vi "equ2hor.vi"(4 "deltat":dbl[unit], 5 "TimeStamp [UT]":timestamp format="%<%H:%M:%S%6u\n%Y/%m/%d>T", 6 "error in (no error)":errorcluster, 7 "site_info":T1={"latitude"=0.3460406188465066, "longitude"=-2.713521559899553, "height"=4123.0, "temperature"=0.0, "pressure"=0.0} {"longitude" format="%_10g"; "latitude" format="%_10g"}, 9 "ra/dec":cluster{"ra":dbl[unit], "dec":dbl[unit]} {"dec" format="%_10g"; "ra" format="%_10g"}) -> (0 "error out":errorcluster, 1 "ra/dec (refraction)":cluster{"ra":dbl[unit], "dec":dbl[unit]} {"dec" format="%_10g"; "ra" format="%_10g"}, 3 "az/zd":cluster{"az":dbl[unit], "zd":dbl[unit]})   [LabVIEW 2009]
uses:
  SiteInformation.ctl
  lib/novas-dll.dll
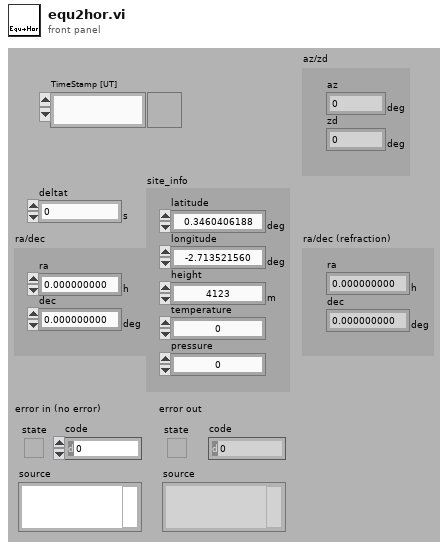
[diagram p1: front panel]
types:
  T1 = typedef "SiteInformation.ctl" = cluster{"latitude":dbl[unit], "longitude":dbl[unit], "height":dbl[unit], "temperature":dbl, "pressure":dbl}
  T2 = cluster{"latitude":dbl, "longitude":dbl, "height":dbl, "temperature":dbl, "pressure":dbl}
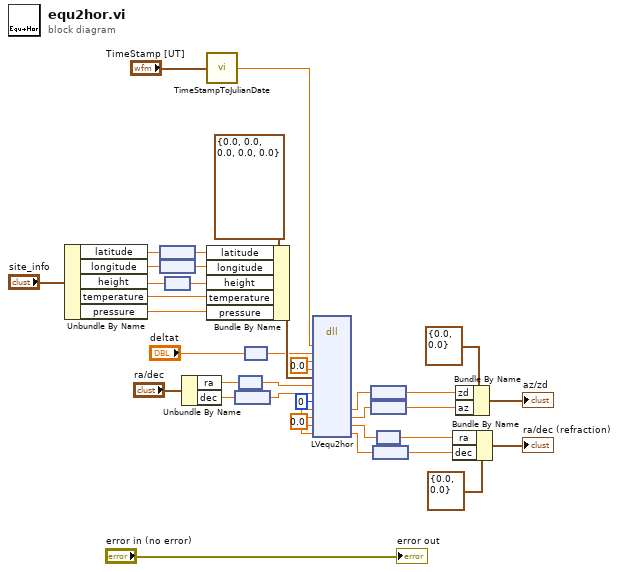
[diagram p0: block diagram]
diagram:
  w28 = 0.0 ("x")
  w35 = 0.0 ("x")
  n1 = Unbundle By Name("site_info") -> ("latitude"=w24:dbl[unit], "longitude"=w23:dbl[unit], "height"=w22:dbl[unit], "temperature"=w21:dbl, "pressure"=w20:dbl)
  n2 = node(w24) -> (w17:dbl)
  n3 = node(w23) -> (w18:dbl)
  n4 = node(w22) -> (w19:dbl)
  n5 = Unbundle By Name("ra/dec") -> ("ra"=w33:dbl[unit], "dec"=w32:dbl[unit])
  n6 = call "TimeStampToJulianDate.vi"("TimeStamp [UT]"="TimeStamp [UT]") -> ("JulianDay"=w2:ext)
  n7 = Bundle By Name(cluster=T2 {"latitude"=0.0, "longitude"=0.0, "height"=0.0, "temperature"=0.0, "pressure"=0.0} ("site_info"), "latitude"=w17, "longitude"=w18, "height"=w19, "temperature"=w21, "pressure"=w20) -> (w15:T2)
  n8 = node(w32) -> (w30:dbl)
  n9 = node(w33) -> (w31:dbl)
  n10 = node("deltat") -> (w14:dbl)
  n11 = dll-call lib="C:/Ohana/LV2009/OhanaOS-LV81/Instruments/Novas/lib/novas-dll.dll" fn="LVequ2hor"("tjd"=w2, "deltat"=w14, "x"=w35, "y"=w35, "site_info"=w15, "ra"=w31, "dec"=w30, "ref_option"=i16 0, "zd"=w28, "az"=w28, "rar"=w28, "decr"=w28) -> ("zd"=w27:dbl, "az"=w26:dbl, "rar"=w3:dbl, "decr"=w9:dbl)  [unwired: 9 in, 5 out]
  n12 = node(w27) -> (w11:dbl[unit])
  n13 = node(w26) -> (w10:dbl[unit])
  n14 = node(w9) -> (w5:dbl[unit])
  n15 = node(w3) -> (w6:dbl[unit])
  n16 = Bundle By Name(cluster=cluster{"ra":dbl[unit], "dec":dbl[unit]} {"ra"=0.0, "dec"=0.0} ("ra/dec (refraction)"), "ra"=w6, "dec"=w5) -> (→"ra/dec (refraction)":cluster{"ra":dbl[unit], "dec":dbl[unit]})
  n17 = Bundle By Name(cluster=cluster{"az":dbl[unit], "zd":dbl[unit]} {"az"=0.0, "zd"=0.0} ("az/zd"), "zd"=w11, "az"=w10) -> (→"az/zd":cluster{"az":dbl[unit], "zd":dbl[unit]})
  "error out" <- "error in (no error)"
